vi "Config Measure Normal.vi"(0 "VISA resource name":refnum<visa-resource-name>, 1 "Element (1: Element 1)":u16(ring)=1 items=["", "Element1", "Element2", "Element3", "Sigma"], 5 "Measure Item (0: V)":u16(ring) items=["V", "A", "W", "VA", "var", "PF", "deg", "V Hz", "A Hz", "Wh", "Wh+", "Wh-", "Ah", "Ah+", "Ah-", "Vpk", "Apk", "Time", "Math"], 7 "State (F: OFF)":bool, 11 "error in (no error)":errorcluster) -> (4 "VISA resource name out":refnum<visa-resource-name>, 15 "error out":errorcluster)   [LabVIEW 2016, in "Yokogawa WT200 Series.lvlib"]
doc: "This VI sends the Normal Measurement Configuration command to the WT200 Series."
uses:
  Yokogawa WT200 Series.lvlib
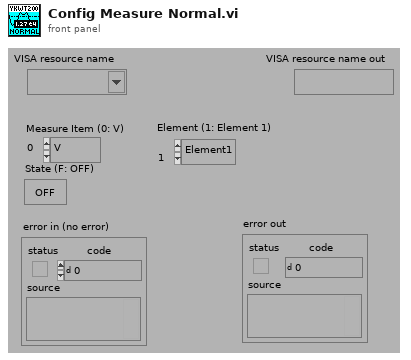
[diagram p1: front panel]
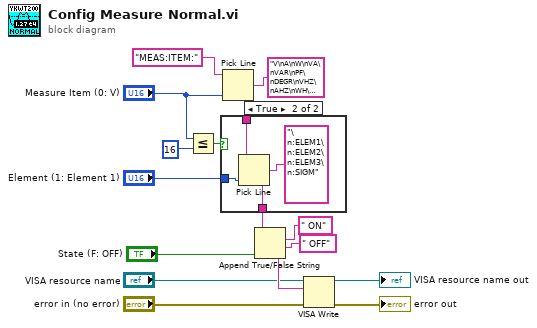
[diagram p0: block diagram]
diagram:
  n1 = Less Or Equal?(x="Measure Item (0: V)", y=u16 16) -> (x <= y?=w7:bool)
  n2 = Pick Line(string ("")="MEAS:ITEM:", multi-line string="V\nA\nW\nVA\nVAR\nPF\nDEGR\nVHZ\nAHZ\nWH\nWHP\nWHM\nAH\nAHP\nAHM\nVPK\nAPK\nTIME\nMATH", line index="Measure Item (0: V)") -> (output string=w12:string)
  n3 = case shown="True" w7 {
    tunnel: w12 -> [w17 w21]
    tunnel: [w17 w20] -> w11
    tunnel: "Element (1: Element 1)" -> [_ w18]
    frame False {
      # "Time or Math"
    }
    frame True {
      n4 = Pick Line(string ("")=w21, multi-line string="\n:ELEM1\n:ELEM2\n:ELEM3\n:SIGM", line index=w18) -> (output string=w20:string)
    }
  }
  n5 = Append True/False String(1:"State (F: OFF)", 2:" OFF", 3:" ON", 4:w11) -> (0:w9:string)
  n6 = VISA Write(VISA resource name="VISA resource name", write buffer=w9, error in (no error)="error in (no error)") -> (VISA resource name out=→"VISA resource name out":refnum<visa-resource-name>, error out=→"error out":errorcluster)  [unwired: 1 out]
